vi "Fit&Smooth Signal.vi"(4 "polynomial order":i32=3, 6 "side points":i32=13, 10 "Signal":dbl[](array[numeric])=[-248.0, -248.0, -244.0, -242.0, -238.0, -239.0, -240.0, -228.0, -228.0, -229.0, -227.0, -223.0, -222.0, -224.0, -221.0, -214.0, -212.0, -208.0, -208.0, -208.0, -202.0, -196.0, -194.0, -198.0, -193.0, -187.0, -184.0, -185.0, -184.0, -178.0, -178.0, -186.0, -193.0, -187.0, -182.0, -178.0, -177.0, -177.0, -175.0, -173.0, -170.0, -173.0, -177.0, -175.0, -177.0, -173.0, -172.0, -171.0, -175.0, -181.0, -182.0, -184.0, -189.0, -186.0, -177.0, -173.0, -181.0, -190.0, -187.0, -179.0, -181.0, -184.0, -186.0, -187.0, -182.0, -176.0, -168.0, -158.0, -152.0, -145.0, -140.0, -135.0, -128.0, -120.0, -116.0, -117.0, -116.0, -112.0, -108.0, -106.0, -98.0, -92.0, -91.0, -94.0, -91.0, -85.0, -83.0, -76.0, -69.0, -70.0, -69.0, -65.0, -66.0, -71.0, -68.0, -66.0, -62.0, -66.0, -66.0, -64.0, -62.0, -70.0, -75.0, -66.0, -65.0, -72.0, -73.0, -73.0, -74.0, -79.0, -85.0, -88.0, -92.0, -91.0, -90.0, -97.0, -102.0, -96.0, -92.0, -92.0, -91.0, -92.0, -82.0, -76.0, -70.0, -70.0, -63.0, -53.0, -47.0, -52.0, -55.0, -44.0, -32.0, -19.0, -16.0, -18.0, -14.0, -7.0, -5.0, -2.0, -4.0, -1.0, 2.0, 5.0, 5.0, -2.0, -10.0, -8.0, -6.0, -5.0, -5.0, -6.0, -8.0, -15.0, -18.0, -16.0, -21.0, -33.0, -35.0, -36.0, -34.0, -34.0, -37.0, -42.0, -44.0, -42.0, -38.0, -32.0, -24.0, -17.0, -12.0, -11.0, -5.0, 4.0, 12.0, 12.0, 9.0, 13.0, 21.0, 22.0, 27.0, 32.0, 35.0, 42.0, 46.0, 44.0, 43.0, 41.0, 44.0, 50.0, 48.0, 43.0, 41.0, 44.0, 45.0, 41.0, 41.0, 32.0, 32.0, 32.0, 30.0, 20.0, 16.0, 11.0, 10.0, 11.0, 8.0, 4.0, 11.0, 13.0, 20.0, 34.0, 44.0, 48.0, 50.0, 53.0, 60.0, 62.0, 65.0, 66.0, 72.0, 80.0, 81.0, 85.0, 81.0, 79.0, 83.0, 84.0, 87.0, 90.0, 89.0, 81.0, 77.0, 75.0, 76.0, 77.0, 72.0, 69.0, 67.0, 61.0, 56.0, 54.0, 50.0, 41.0, 35.0, 40.0, 45.0, 52.0, 62.0, 69.0, 72.0, 75.0, 82.0, 88.0, 86.0, 87.0, 97.0, 104.0, 110.0, 112.0, 112.0, 112.0, 117.0, 120.0, 116.0, 114.0, 113.0, 113.0, 120.0, 118.0, 114.0, 116.0, 115.0, 115.0, 108.0, 99.0, 93.0, 89.0, 88.0, 83.0, 80.0, 85.0, 93.0, 97.0, 100.0, 104.0, 113.0, 122.0, 134.0, 135.0, 136.0, 134.0, 143.0, 147.0, 151.0, 151.0, 154.0, 155.0, 158.0, 162.0, 161.0, 155.0, 150.0, 152.0, 157.0, 162.0, 158.0, 156.0, 148.0, 145.0, 142.0, 138.0, 134.0, 135.0, 137.0, 136.0, 131.0, 133.0, 144.0, 161.0, 165.0, 169.0, 172.0, 177.0, 184.0, 191.0, 194.0, 197.0, 200.0, 202.0, 200.0, 201.0, 200.0, 200.0, 199.0, 199.0, 201.0, 199.0, 194.0, 189.0, 183.0, 176.0, 174.0, 174.0, 171.0, 170.0, 168.0, 171.0, 179.0, 188.0, 196.0, 204.0, 210.0, 218.0, 222.0, 224.0, 231.0, 231.0, 232.0, 234.0, 241.0, 250.0, 251.0, 248.0, 246.0, 246.0, 249.0, 249.0, 243.0, 243.0, 241.0, 237.0, 233.0, 234.0, 226.0, 219.0, 221.0, 223.0, 226.0, 235.0, 245.0, 261.0, 274.0, 278.0, 276.0, 278.0, 283.0, 287.0, 297.0, 302.0, 301.0, 295.0, 299.0, 299.0, 294.0, 290.0, 291.0, 290.0, 287.0, 288.0, 285.0, 284.0, 276.0, 269.0, 271.0, 273.0, 280.0, 290.0, 298.0, 308.0, 318.0, 319.0, 319.0, 330.0, 335.0, 337.0, 341.0, 348.0, 348.0, 348.0, 350.0, 354.0, 351.0, 356.0, 355.0, 350.0, 351.0, 344.0, 336.0, 332.0, 330.0, 332.0, 335.0, 343.0, 358.0, 361.0, 370.0, 378.0, 384.0, 397.0, 403.0, 405.0, 404.0, 407.0, 410.0, 408.0, 409.0, 414.0, 417.0, 414.0, 409.0, 405.0, 405.0, 399.0, 391.0, 387.0, 392.0, 399.0, 405.0, 417.0, 418.0, 427.0, 438.0, 447.0, 450.0, 456.0, 463.0, 466.0, 469.0, 466.0, 468.0, 470.0, 471.0, 473.0, 472.0, 474.0, 473.0, 468.0, 462.0, 452.0, 457.0, 468.0, 479.0, 490.0, 496.0, 502.0, 505.0, 519.0, 525.0, 528.0, 527.0, 530.0, 536.0, 537.0, 535.0, 528.0, 531.0, 526.0, 521.0, 524.0, 524.0, 520.0, 524.0, 536.0, 552.0, 561.0, 570.0, 572.0, 580.0, 584.0, 588.0, 588.0]) -> (2 "SmoothFitSignal":dbl[](graph))   [LabVIEW 2014]
uses:
  <vilib>/Analysis/3filter.llb/Savitzky-Golay Filter (DBL).vi
  <vilib>/imath/engines/lvmath2/RunTimeEngine/RangeToken/NIMS_Range.vi
  <instcachedir>/0/NIMS_Range_9BCE657718DF4976A877346C61F22738.lvgen/NIMS_Range_9BCE657718DF4976A877346C61F22738_001.vi
  <vilib>/imathl/engines/lvmath/Functions/Error Handling/Create Error.vi
  <vilib>/imath/engines/lvmath2/RunTimeEngine/BuiltInFunctions/polyfit/NIMS_[2o]_polyfit.vi
  <vilib>/imath/engines/lvmath2/RunTimeEngine/ErrorHandling/NIMS_Error From Error Code.vi
  <vilib>/imath/engines/lvmath2/RunTimeEngine/BuiltInFunctions/polyval/NIMS_polyval(GV,GM).vi
  <instcachedir>/0/NIMS_polyval(GV,GM)_E12556DC54744E0C81968744501C4F35.lvgen/NIMS_polyval(GV,GM)_E12556DC54744E0C81968744501C4F35_002.vi
  <vilib>/imath/engines/lvmath2/RunTimeEngine/ArithmeticOperatorToken/NIMS_ArithmeticOperator_minus.vi
  <instcachedir>/0/NIMS_ArithmeticOperator_minus_39C0593E74DA4138ACA2AB742906488D.lvgen/NIMS_ArithmeticOperator_minus_39C0593E74DA4138ACA2AB742906488D_003.vi
  <vilib>/imath/engines/lvmath2/RunTimeEngine/NodeEndStatement/NIMS_NodeEndStatement_Output.vi
  <instcachedir>/0/NIMS_NodeEndStatement_Output_53EC0D466D134D7ABD903AC30B43404B.lvgen/NIMS_NodeEndStatement_Output_53EC0D466D134D7ABD903AC30B43404B_005.vi
  <vilib>/imath/engines/lvmath2/RunTimeEngine/ErrorHandling/NIMS_Finalize Error.vi
  <vilib>/Analysis/NI_AALBase.lvlib
panel:
  out "FitSignal":dbl[](graph)
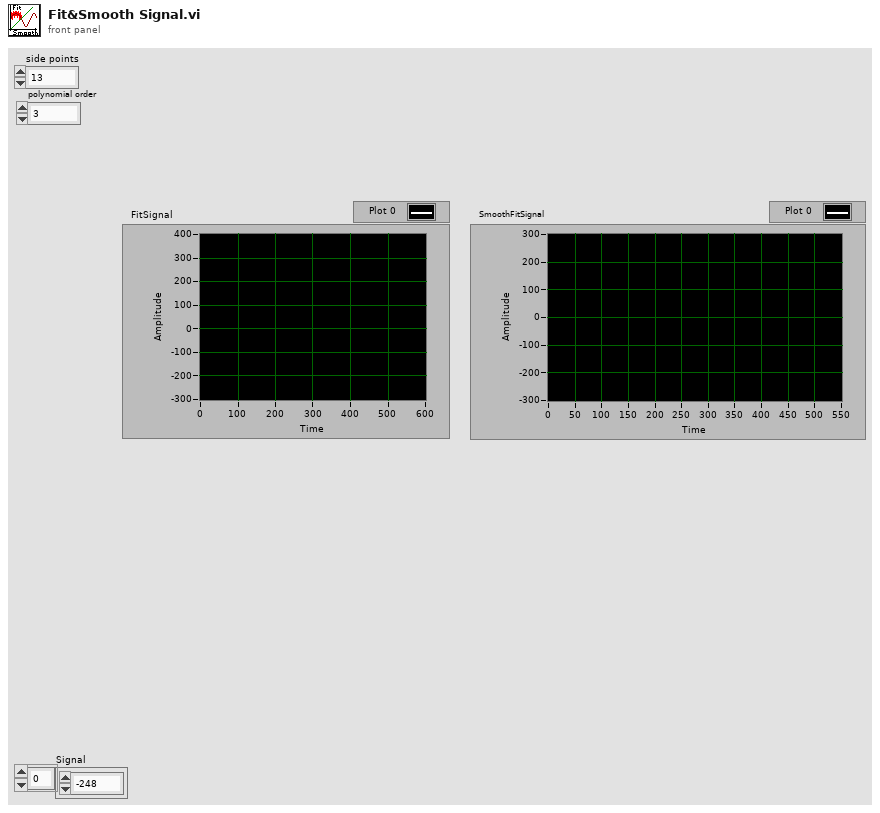
[diagram p1: front panel]
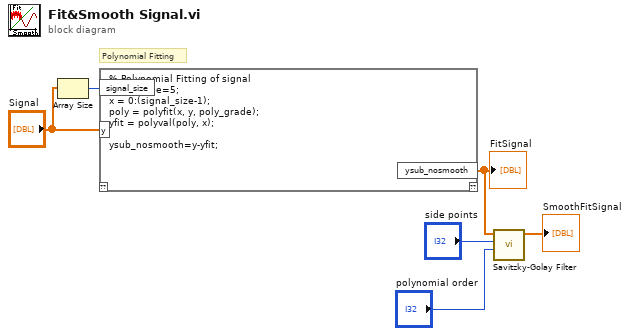
[diagram p0: block diagram]
diagram:
  # "Polynomial Fitting"
  n1 = Array Size(array="Signal") -> (size(s)=w6:i32)
  n2 = mathscript code="% Polynomial Fitting of signal\npoly_grade=5;\nx = 0:(signal_size-1);\npoly = polyfit(x, y, poly_grade); \nyfit = polyval(poly, x); \n\nysub_nosmooth=y-yfit;"("signal_size"=w6, "y"="Signal") -> ("ysub_nosmooth"=w3:dbl[])  [unwired: 1 in, 1 out]
  "FitSignal" <- w3
  n3 = call-poly <vilib>:"Savitzky-Golay Filter.vi"("polynomial order"="polynomial order", "side points"="side points", "X"=w3) -> ("Filtered X"=→"SmoothFitSignal":dbl[])  [unwired: 7 in, 1 out]
